vi "driveLogic.vi"(9 "Axes 2":dbl[](array[numeric]), 10 "Axes":dbl[](array[numeric]), 11 "Cluster in":cluster{bool, "Numeric":i32}) -> (3 "Cluster out":T1)   [LabVIEW 2014]
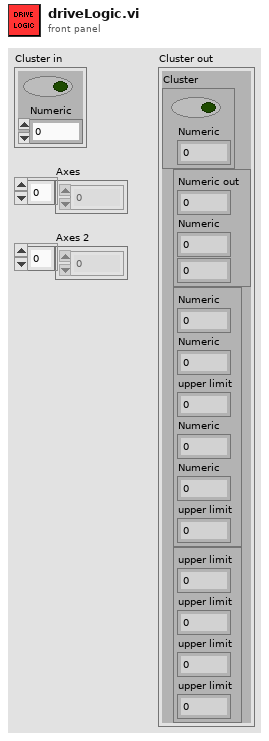
[diagram p1: front panel]
types:
  T1 = cluster{"Cluster":cluster{bool, "Numeric":i32}, cluster{"Numeric out":dbl, "Numeric":dbl, dbl}, cluster{"Numeric":dbl, "Numeric":dbl, "upper limit":dbl, "Numeric":dbl, "Numeric":dbl, "upper limit":dbl}, cluster{"upper limit":dbl, "upper limit":dbl, "upper limit":dbl, "upper limit":dbl}}
  T2 = cluster{"upper limit":dbl, "upper limit":dbl, "upper limit":dbl, "upper limit":dbl}
  T3 = cluster{"Numeric":dbl, "Numeric":dbl, "upper limit":dbl, "Numeric":dbl, "Numeric":dbl, "upper limit":dbl}
  T4 = cluster{"Cluster in":cluster{bool, "Numeric":i32}, cluster{"Numeric out":dbl, "Numeric":dbl, dbl}, cluster{"Numeric":dbl, "Numeric":dbl, "upper limit":dbl, "Numeric":dbl, "Numeric":dbl, "upper limit":dbl}, cluster{"upper limit":dbl, "upper limit":dbl, "upper limit":dbl, "upper limit":dbl}}
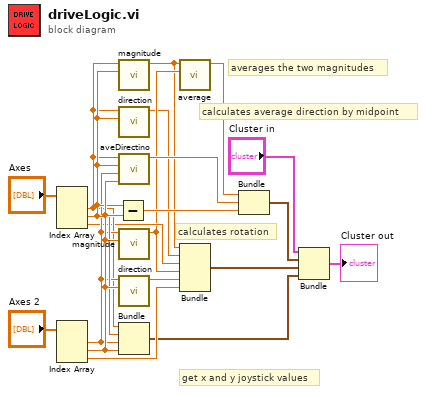
[diagram p0: block diagram]
diagram:
  # "get x and y joystick values"
  # "calculates rotation"
  # "calculates average direction by midpoint"
  # "averages the two magnitudes"
  n1 = Index Array(array="Axes") -> (element #1=w15:dbl, element #2=w17:dbl, element #3=w12:dbl)  [unwired: 3 in]
  n2 = Index Array(array="Axes 2") -> (element #1=w16:dbl, element #2=w19:dbl, element #3=w13:dbl)  [unwired: 3 in]
  n3 = Subtract(x=w17, y=w19) -> (x-y=w14:dbl)
  n4 = call "magnitude.vi"("upper limit"=w17, "upper limit 2"=w15) -> ("Numeric"=w9:dbl)  [unwired: 9 in]
  n5 = call "direction.vi"("upper limit"=w17, "upper limit 2"=w15) -> ("Numeric"=w7:dbl)  [unwired: 9 in]
  n6 = call "aveDirectino.vi"("upper limit"=w19, "upper limit 3"=w16, "upper limit 2"=w17, "upper limit 4"=w15) -> ("Numeric"=w18:dbl)  [unwired: 7 in]
  n7 = call "magnitude.vi"("upper limit"=w19, "upper limit 2"=w16) -> ("Numeric"=w10:dbl)  [unwired: 9 in]
  n8 = call "direction.vi"("upper limit"=w19, "upper limit 2"=w16) -> ("Numeric"=w8:dbl)  [unwired: 9 in]
  n9 = Bundle("upper limit"=w15, "upper limit"=w17, "upper limit"=w16, "upper limit"=w19) -> (w5:T2)  [unwired: 1 in]
  n10 = call "average.vi"("Numeric in"=w10, "Numeric 3"=w9) -> ("Numeric out"=w11:dbl)  [unwired: 9 in]
  n11 = Bundle("Numeric"=w9, "Numeric"=w7, "upper limit"=w12, "Numeric"=w10, "Numeric"=w8, "upper limit"=w13) -> (w4:T3)  [unwired: 1 in]
  n12 = Bundle("Numeric out"=w11, "Numeric"=w18, w14) -> (w3:cluster{"Numeric out":dbl, "Numeric":dbl, dbl})  [unwired: 1 in]
  n13 = Bundle("Cluster in"="Cluster in", w3, w4, w5) -> (→"Cluster out":T4)  [unwired: 1 in]
